vi "Close_Connection.vi"() -> (2 "Connection Closed":bool)   [LabVIEW 2015]
uses:
  CryoTUM-V1.0/Instrument_Setup.vi
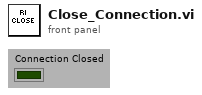
[diagram p1: front panel]
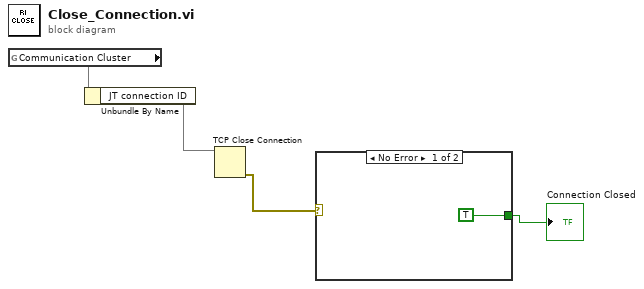
[diagram p0: block diagram]
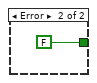
[diagram p2: hidden frame]
diagram:
  n1 = global read "Instrument_Setup.vi" "Communication Cluster"() -> (w3)
  n2 = Unbundle By Name(w3) -> ("JT connection ID"=w4)
  n3 = TCP Close Connection(connection ID=w4) -> (error out=w2:errorcluster)  [unwired: 2 in, 1 out]
  n4 = case shown="No Error" w2 {
    tunnel: [TRUE FALSE] -> w1
    frame No Error {
    }
    frame Error {
    }
  }
  "Connection Closed" <- w1
